vi "TestFollowWall.vi"() -> ()   [LabVIEW 2016]
uses:
  <vilib>/Platform/TimedLoop/XDataNode/XDataNode.xnode
  <vilib>/Platform/TimedLoop/XDataNode/nitl_modes.ctl
  <vilib>/Platform/TimedLoop/XDataNode/XDNodeRunTimeDep.lvlib
  <vilib>/Platform/TimedLoop/XDataNode/wakeup.ctl
  <vilib>/Platform/TimedLoop/XDataNode/timing_clust.ctl
  <vilib>/robotics/Steering/Steering Frame/NI_Robotics_Steering Frame.lvclass
  <vilib>/robotics/Steering/Steering Frame/Apply Steering Frame Velocity to Wheels.vi
  <vilib>/myRIO/Instrument Drivers/Utilities/Utilities.lvlib
  <vilib>/robotics/Steering/Differential Steering Frame/NI_Robotics_Differential Steering Frame.lvclass
  C:/Program Files (x86)/National Instruments/LabVIEW 2016/vi.lib/robotics/Steering/Special Steering Frame/NI_Robotics_Special Steering Frame.lvclass
  C:/Program Files (x86)/National Instruments/LabVIEW 2016/vi.lib/robotics/Steering/Steering Frame/NI_Robotics_Steering Frame.lvclass
  <vilib>/robotics/Steering/Wheel/Rotation Direction.ctl
  <vilib>/robotics/Steering/Wheel/NI_Robotics_Wheel.lvclass
  <vilib>/robotics/Steering/Wheel/Wheel Parameters.ctl
  MotorControl/Configurations.ctl
  <vilib>/robotics/Steering/Wheel/Wheel State.ctl
panel:
  out "Robot Position":cluster{dbl[], dbl[]}(graph)
  in  "stop":bool
  in  "Start":bool
  out "calculated wheel states":T1[](array[typedef])
  out "ir distances rf":dbl[][](array[numeric])
  out "ir distances":dbl[](array[numeric])
  in  "Robot Configuration":T2={"wheel parameters"={"wheel radius"=0.05, "gear ratio"=1.0, "forward rotation direction"=0}, "wheel separation"=0.19, "Encoder Pulse Per Rev"=1856.0, "Update Period (sec)"=20.0, "Initial posture frame"=[0.0, 0.0, 0.0]} {"wheel parameters"."forward rotation direction" items=["Clockwise", "Counterclockwise"]}
  out "dt":dbl
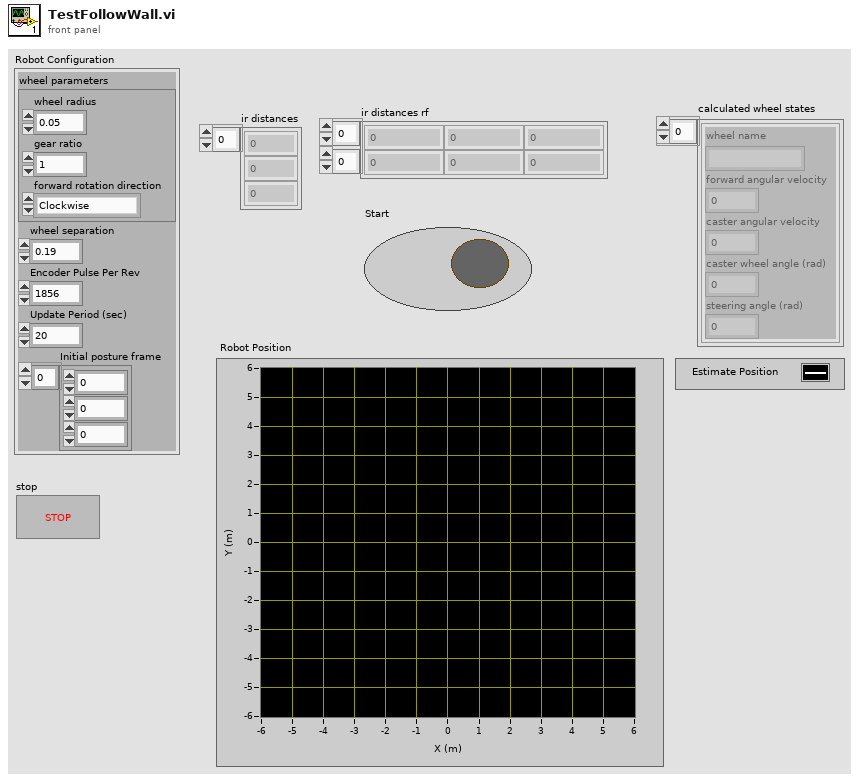
[diagram p1: front panel]
types:
  T1 = typedef "NI_Robotics_Wheel.lvclass/Wheel State.ctl" = cluster{"wheel name":string, "forward angular velocity":dbl, "caster angular velocity":dbl, "caster wheel angle (rad)":dbl, "steering angle (rad)":dbl}
  T2 = typedef "Configurations.ctl" = cluster{"wheel parameters":T3, "wheel separation":dbl, "Encoder Pulse Per Rev":dbl, "Update Period (sec)":dbl, "Initial posture frame":dbl[]}
  T3 = typedef "NI_Robotics_Wheel.lvclass/Wheel Parameters.ctl" = cluster{"wheel radius":dbl, "gear ratio":dbl, "forward rotation direction":T4}
  T4 = typedef "NI_Robotics_Wheel.lvclass/Rotation Direction.ctl" = u16
  T5 = typedef "MotorObject.ctl" = cluster{"PWM Motor Left":T6, "PWM Motor Right":T6, "DIR Motor Left":T13, "Encoder Motor Left":T16, "Encoder Motor Right":T16, "DIR Motor Right":T13, "Left DIR Forward":bool}
  T6 = typedef "PWM.lvlib/PWM Reference.ctl" = cluster{"myRIO Reference":T7, "PWM Channels Enum":T11, "PWM Configuration":T12}
  T7 = typedef "myRIO Generic Hardware Reference.ctl" = cluster{"myRIO Model":T8, "myRIO Hardware Reference":T9}
  T8 = typedef "Hardware Version Enum.ctl" = enum16{"Unknown", "myRIO-1900", "myRIO-1950", "roboRIO", "NI ELVIS RIO CM"}
  T9 = typedef "myRIO v1.0 Reference.ctl" = cluster{"Generic FPGA Reference":T10, "Allow multiple opens":bool}
  T10 = typedef "Generic FPGA Reference.ctl" = refnum<k20>
  T11 = typedef "PWM Channels Enum.ctl" = enum16{"Not Connected", "C/PWM0", "C/PWM1", "A/PWM0", "A/PWM1", "A/PWM2", "B/PWM0", "B/PWM1", "B/PWM2", "PWM/PWM0", "PWM/PWM1", "PWM/PWM2", "PWM/PWM3", "PWM/PWM4", "PWM/PWM5", "PWM/PWM6", "PWM/PWM7", "PWM/PWM8", "PWM/PWM9"}
  T12 = typedef "PWM.lvlib/PWM Configuration.ctl" = cluster{"Frequency":dbl, "Duty Cycle":dbl}
  T13 = typedef "DIO.lvlib/DIO Reference.ctl" = cluster{"myRIO Reference":T7, "DIO Channels List":T14}
  T14 = typedef "DIO Channels List.ctl" = T15[]
  T15 = typedef "DIO Channels Enum.ctl" = enum16{"Not Connected", "C/DIO0", "C/DIO1", "C/DIO2", "C/DIO3", "C/DIO4", "C/DIO5", "C/DIO6", "C/DIO7", "A/DIO0", "A/DIO1", "A/DIO2", "A/DIO3", "A/DIO4", "A/DIO5", "A/DIO6", "A/DIO7", "A/DIO8", "A/DIO9", "A/DIO10", "A/DIO11", "A/DIO12", "A/DIO13", "A/DIO14", "A/DIO15", "B/DIO0", "B/DIO1", "B/DIO2", "B/DIO3", "B/DIO4", "B/DIO5", "B/DIO6", "B/DIO7", "B/DIO8", "B/DIO9", "B/DIO10", "B/DIO11", "B/DIO12", "B/DIO13", "B/DIO14", "B/DIO15", "LED0", "LED1", "LED2", "LED3", "Button0", "DIO/DIO0", "DIO/DIO1", "DIO/DIO2", "DIO/DIO3", "DIO/DIO4", "DIO/DIO5", "DIO/DIO6", "DIO/DIO7", "DIO/DIO8", "DIO/DIO9", "SPI/CS0", "SPI/CS1", "SPI/CS2", "SPI/CS3", "LED RADIO (Green)", "LED RADIO (Red)", "LED COMM (Green)", "LED COMM (Red)", "LED MODE (Green)", "LED MODE (Red)"}
  T16 = typedef "Encoder.lvlib/Encoder Reference.ctl" = cluster{"myRIO Reference":T7, "Encoder Channels Enum":T17}
  T17 = typedef "Encoder Channels Enum.ctl" = enum16{"Not Connected", "C/ENC0", "C/ENC1", "A/ENC", "B/ENC", "DIO/ENC0", "DIO/ENC1", "DIO/ENC2", "DIO/ENC3", "DIO/ENC4"}
  T18 = typedef "Measurement Parameters.ctl" = cluster{"Start Step":u32, "End Step":u32, "Cluster Count":u32, "Scan Interval":u32, "Number of Scans":u32, "Measurement Type":T19}
  T19 = typedef "Measurement Type.ctl" = enum16{"MS"}
  T20 = typedef "XDNodeRunTimeDep.lvlib/timing_clust.ctl" = cluster{"Expected End [f-1]":u64, "Actual End [f-1]":u64, "Finished Late? [f-1]":bool, "Expected End [i-1]":u64, "Actual End [i-1]":u64, "Finished Late? [i-1]":bool, "Expected Start [i]":u64, "Actual Start [i]":u64, "Expected Start [f]":u64, "Actual Start [f]":u64, "Source Name":string, "Structure Name":string, "Period":i64, "Deadline":i64, "Offset":i64, "Start":i64, "Priority":i32, "Timeout":i32, "Mode":T21, "Wakeup Reason":T22, "Error":errorcluster, "Source Type":string, "Secondary Source Type":string, "Global End Time":u64, "Global Start Time":u64, "Frame Duration":u64, "Iteration Duration":u64, "Assigned CPU":i32, "I/O Scan Engine Mode":u32}
  T21 = typedef "XDNodeRunTimeDep.lvlib/nitl_modes.ctl" = enum32{"No Change", "Process missed periods, maintain original phase", "Discard missed periods, maintain original phase", "Process missed periods, ignore original phase", "Discard missed periods, ignore original phase"}
  T22 = typedef "XDNodeRunTimeDep.lvlib/wakeup.ctl" = enum32{"Normal", "Aborted", "Asynchronous wakeup", "Timing source error", "Timed loop error", "Timeout"}
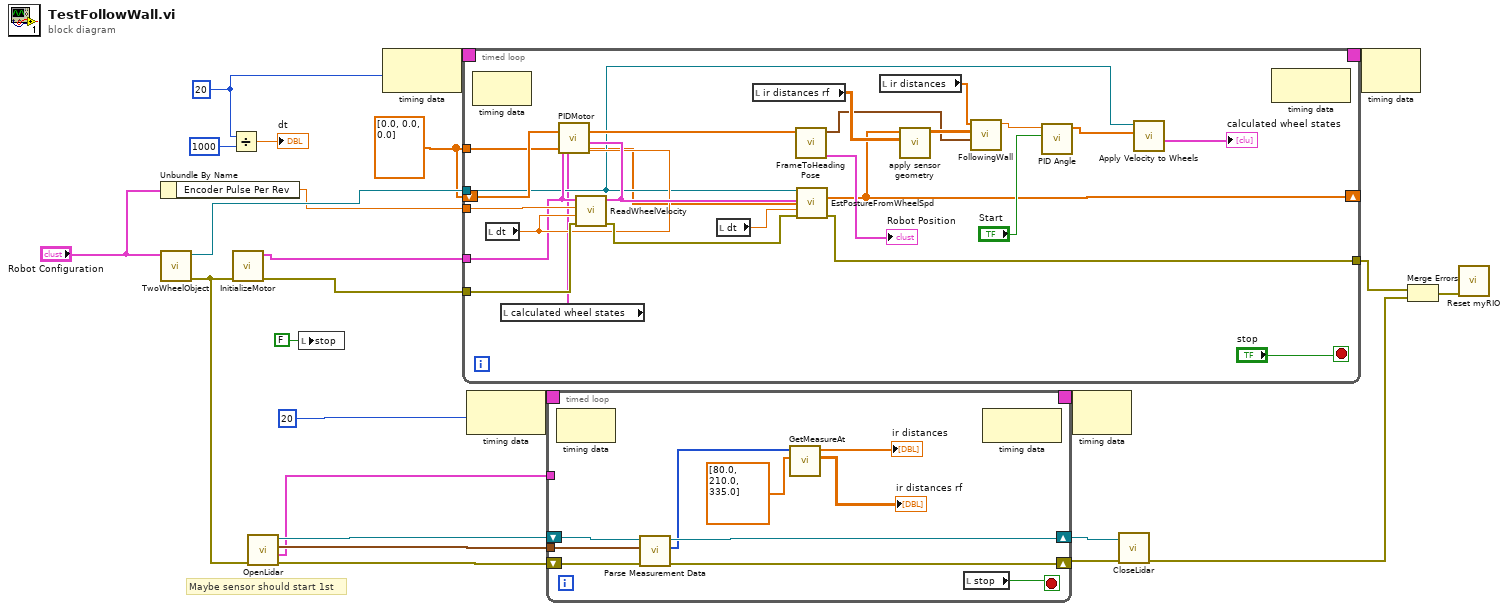
[diagram p0: block diagram]
diagram:
  w5 = dbl[] [0.0, 0.0, 0.0] ("initial posture")
  w23 = i64 20 ("Period")
  # "Maybe sensor should start 1st"
  n1 = Unbundle By Name("Robot Configuration") -> ("Encoder Pulse Per Rev"=w7:dbl)
  n2 = call "TwoWheelObject.vi"("Robot Configuration"="Robot Configuration") -> ("error out"=w8:errorcluster, "differential steering frame out"=w17:refnum<class "NI_Robotics_Differential Steering Frame.lvclass">)  [unwired: 9 in]
  n3 = Divide(x=w23, y=i64 1000) -> (x/y=→"dt":dbl)
  n4 = call "InitializeMotor.vi"("error in"=w8) -> ("error out"=w18:errorcluster, "Motor Ref"=w19:T5)  [unwired: 9 in]
  n5 = call "OpenLidar.vi"("error in (no error)"=w8) -> ("error out"=w13:errorcluster, "Params Out"=w9:cluster{"angle":dbl[], "id":i32[], "kk":dbl[]}, "Measurement Parameters"=w11:T18, "VISA Refnum out"=w14:refnum<visa-resource-name>)  [unwired: 7 in]
  n6 = local write "stop"(FALSE ("stop")) -> ()
  n7 = node-c288(w23) -> (w25:T20)
  n8 = timed-loop {
    timing: w25 -> [_]
    timing-out: [_] -> w24
    tunnel: w19 -> [w38]
    tunnel: w18 -> [w48]
    tunnel: w17 -> [w37]
    shift-right: [w29] -> _
    shift-left: w5 -> [w44]
    tunnel: w7 -> [w40]
    tunnel: w5 -> [w33]
    tunnel: [w26] -> w2
    stop <- "stop" stop-if-true
    n9 = node-c288() -> ()  [unwired: 1 in, 1 out]
    n10 = local read "dt"() -> (w39:dbl)
    n11 = local read "calculated wheel states"() -> (w35:T1[])
    n12 = call "ReadWheelVelocity.vi"("error in"=w48, 9:w39, "Robot Configuration"=w40, "Motor Ref"=w38) -> ("error out"=w45:errorcluster, "Motor Ref"=w47:T5)  [unwired: 5 in, 1 out]
    n13 = call "PIDMotor.vi"("Motor Object"=w38, "Robot Configuration"=w35, "calculated wheel states"=w47, "Wheel Velocity"=w39) -> ()  [unwired: 7 in]
    n14 = local read "dt"() -> (w46:dbl)
    n15 = local read "ir distances rf"() -> (w43:dbl[][])
    n16 = call "FrameToHeadingPose.vi"("Posture In"=w44) -> ("Robot Vector"=→"Robot Position":cluster{"Array":dbl[], "Array":dbl[]}, "Heading Frame"=w27:cluster{"X":sgl, "Y":sgl, "theta":dbl})  [unwired: 7 in, 2 out]
    n17 = call "EstPostureFromWheelSpd.vi"("differential steering frame in"=w37, "Wheel Velocity"=w47, "Robot Configuration"=w33, 9:w46, "error in (no error)"=w45) -> ("estimated steering frame posture"=w29:dbl[], "error out"=w26:errorcluster)  [unwired: 8 in, 1 out]
    n18 = local read "ir distances"() -> (w41:dbl[])
    n19 = call "apply sensor geometry.vi"("Posture In"=w43, "IF readings\n(meters)"=w29) -> ("ir distances wf"=w42:dbl[][])  [unwired: 9 in]
    n20 = call "FollowingWall.vi"("Heading Frame"=w27, "ir distances wf"=w42, "ir distances"=w41) -> ("theta_error"=w28:dbl)  [unwired: 8 in]
    n21 = call "PID Angle.vi"("Enable?"="Start", "Angle to Goal"=w28) -> ("Frame Velocity"=w31:dbl[])  [unwired: 9 in]
    n22 = call-poly <vilib>:"Apply Velocity to Wheels.vi"("steering frame velocity"=w31, "steering frame in"=w37) -> ("calculated wheel states"=→"calculated wheel states":T1[])  [unwired: 6 in, 3 out]
    n23 = node-c288() -> ()  [unwired: 1 in, 1 out]
  }
  n24 = node-c288(i64 20 ("Period")) -> (w16:T20)
  n25 = timed-loop {
    tunnel: w11 -> [w60]
    shift-right: [w56] -> w12
    shift-left: w14 -> [w59]
    shift-right: [w57] -> w4
    shift-left: w13 -> [w58]
    timing: w16 -> [_]
    timing-out: [_] -> w15
    tunnel: w9 -> [_]
    stop <- w52 stop-if-true
    n26 = node-c288() -> ()  [unwired: 1 in, 1 out]
    n27 = call "Parse Measurement Data.vi"("error in (no error)"=w58, "Measurement Parameters"=w60, "VISA Refnum in"=w59) -> ("error out"=w57:errorcluster, "Measurement Data"=w55:i32[], "VISA Refnum out"=w56:refnum<visa-resource-name>)  [unwired: 6 in]
    n28 = call "GetMeasureAt.vi"("Sub Index"=dbl[] [80.0, 210.0, 335.0], "Measurement Data"=w55) -> ("ir distances rf"=→"ir distances rf":dbl[][], "ir distances"=→"ir distances":dbl[])  [unwired: 8 in]
    n29 = local read "stop"() -> (w52:bool)
    n30 = node-c288() -> ()  [unwired: 1 in, 1 out]
  }
  n31 = node-c288(w15) -> ()  [unwired: 1 out]
  n32 = call "CloseLidar.vi"("error in (no error)"=w4, "VISA Refnum in"=w12) -> ("error out"=w3:errorcluster)  [unwired: 9 in]
  n33 = node-c288(w24) -> ()  [unwired: 1 out]
  n34 = Merge Errors(w2, w3) -> (w1:errorcluster)
  n35 = call <vilib>:"Reset myRIO.vi"("error in (no error)"=w1) -> ()  [unwired: 10 in, 1 out]
